vi "remove point.vi"(5 "Overwrite Lib Path":path, 8 "error in (no error)":errorcluster, 10 "point_id":u32, 11 "index_ptr":u64) -> (0 "error out":errorcluster, 3 "index_ptr out":u64)   [LabVIEW 2020, in "KD Tree.lvlib"]
doc: "FLANN_EXPORT int flann_remove_point(flann_index_t index_ptr,\n unsigned int point_id);"
uses:
  KD Tree.lvlib
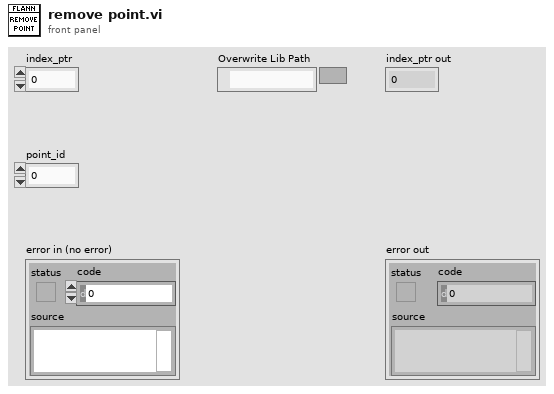
[diagram p1: front panel]
types:
  T1 = typedef "Semaphore RefNum" = refnum<k1>
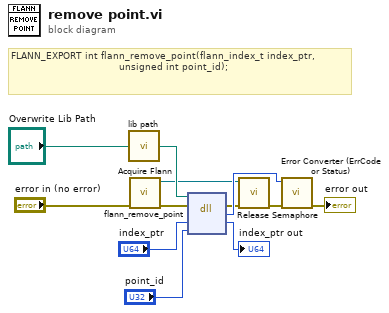
[diagram p0: block diagram]
diagram:
  # "FLANN_EXPORT int flann_remove_point(flann_index_t index_ptr,\n                                    unsigned int point_id);"
  n1 = call "lib path.vi"("Overwrite Lib Path"="Overwrite Lib Path") -> ("lib path"=w5:path)
  n2 = call "Acquire Flann.vi"("error in (no error)"="error in (no error)") -> ("error out"=w3:errorcluster, "semaphore"=w1:T1)  [unwired: 9 in]
  n3 = dll-call lib="E:/Labview/LV 2020/Libs/flann/flann.*" fn="flann_remove_point"(path in=w5, error in=w3, "index_ptr"="index_ptr", "point_id"="point_id") -> (error out=w7:errorcluster, "return type"=w12:i32, "index_ptr"=→"index_ptr out":u64)  [unwired: 2 in, 1 out]
  n4 = call <vilib>:"Release Semaphore.vi"("error in (no error)"=w7, "semaphore"=w1) -> ("error out"=w2:errorcluster)  [unwired: 4 in, 1 out]
  n5 = call "Error Converter (ErrCode or Status).vi"("error in (no error)"=w2, "error code"=w12) -> ("error out"=→"error out":errorcluster)  [unwired: 9 in]
